vi "SetNumStages.vi"(8 "error in":errorcluster, 10 "#Stages":enum16{"None", "1 Pole", "2 Pole"}(ring), 11 "Port":refnum<visa-resource-name>) -> (0 "error out":errorcluster, 3 "Port out":refnum<visa-resource-name>)   [LabVIEW 2018]
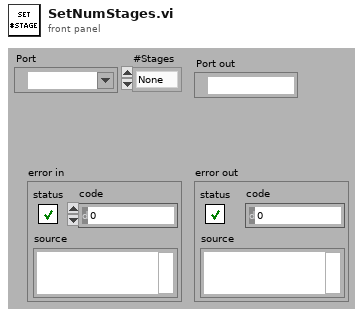
[diagram p1: front panel]
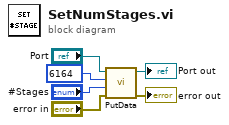
[diagram p0: block diagram]
diagram:
  n1 = call "PutData.vi"("error in"="error in", "Value"="#Stages", "Location"=u32 6164, "Port"="Port") -> ("error out"=→"error out":errorcluster, "Port out"=→"Port out":refnum<visa-resource-name>)  [unwired: 6 in]
